vi "실습 5-1 클러스터 풀기와 묶기.vi"() -> ()   [LabVIEW 2014]
panel:
  out "클러스터 4":T1
  in  "클러스터 3":T1
  out "클러스터 2":T1
  in  "클러스터":T1
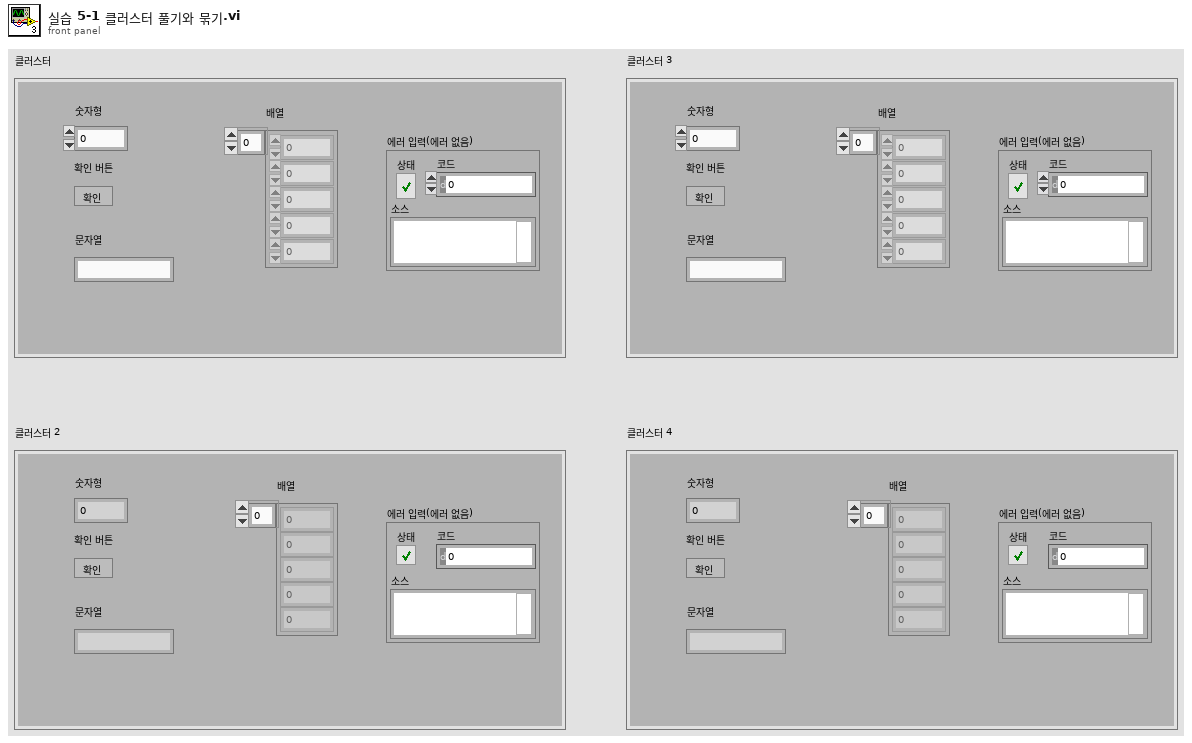
[diagram p1: front panel]
types:
  T1 = cluster{"숫자형":dbl, "확인 버튼":bool, "문자열":string, "배열":dbl[], "error in (no error)":errorcluster}
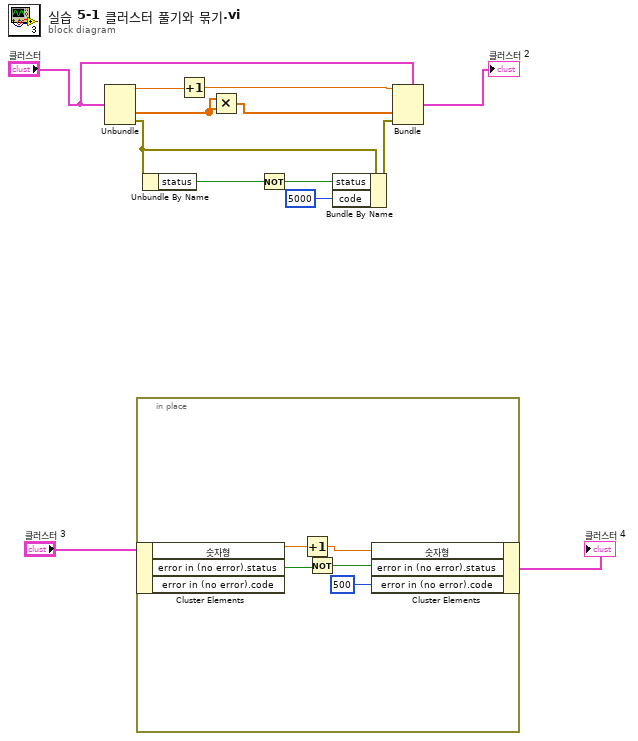
[diagram p0: block diagram]
diagram:
  n1 = Unbundle("클러스터") -> ("숫자형"=w11:dbl, "배열"=w4:dbl[], "error in (no error)"=w9:errorcluster)  [unwired: 2 out]
  n2 = in-place {
    n3 = in-place-cluster #1("클러스터 3") -> ("숫자형"=w18:dbl, "error in (no error).status"=w16:bool)  [unwired: 1 out]
    n4 = Increment(x=w18) -> (x+1=w17:dbl)
    n5 = Not(x=w16) -> (.not. x?=w15:bool)
    n6 = in-place-cluster #1("숫자형"=w17, "error in (no error).status"=w15, "error in (no error).code"=500) -> (→"클러스터 4":T1)
  }
  n7 = Unbundle By Name(w9) -> ("status"=w8:bool)
  n8 = Increment(x=w11) -> (x+1=w10:dbl)
  n9 = Multiply(x=w4, y=w4) -> (x*y=w3:dbl[])
  n10 = Not(x=w8) -> (.not. x?=w7:bool)
  n11 = Bundle By Name(cluster=w9, "status"=w7, "code"=5000) -> (w6:errorcluster)
  n12 = Bundle(cluster="클러스터", "숫자형"=w10, "배열"=w3, "error in (no error)"=w6) -> (→"클러스터 2":T1)  [unwired: 2 in]
